vi "ReadTxBuffer.vi"(8 "error in":errorcluster, 11 "VISA Refnum in":refnum<visa-resource-name>) -> (0 "error out":errorcluster, 1 "Tx Buffer":string, 2 "Tx Buffer Len":string, 3 "VISA Refnum out":refnum<visa-resource-name>)   [LabVIEW 2020]
panel:
  out "tx_len":u32
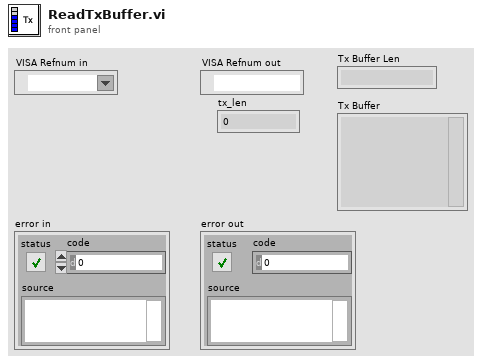
[diagram p1: front panel]
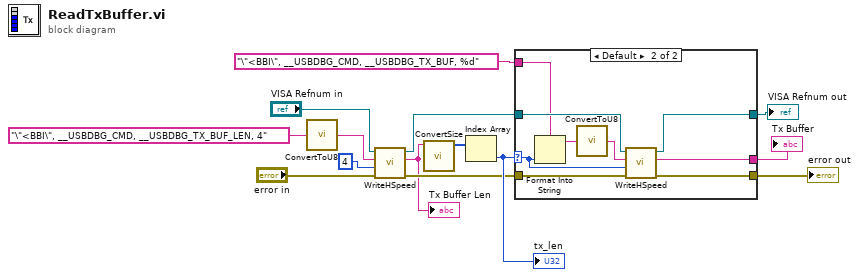
[diagram p0: block diagram]
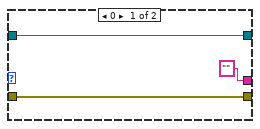
[diagram p2: hidden frame]
diagram:
  n1 = call "ConvertToU8.vi"("struct"="\"<BBI\", __USBDBG_CMD, __USBDBG_TX_BUF_LEN, 4" ("write buffer")) -> ("Binary"=w12:string)
  n2 = call "WriteHSpeed.vi"("error in"="error in", "Reply length"=4, "write buffer"=w12, "VISA Refnum in"="VISA Refnum in") -> ("error out"=w8:errorcluster, "read buffer"=w4:string, "VISA Refnum out"=w6:refnum<visa-resource-name>)  [unwired: 5 in]
  "Tx Buffer Len" <- w4
  n3 = call "ConvertSize.vi"("read buffer"=w4) -> ("size()"=w5:u32[])  [unwired: 9 in, 1 out]
  n4 = Index Array(array=w5) -> (element=w14:u32)  [unwired: 1 in]
  "tx_len" <- w14
  n5 = case shown="Default" w14 {
    selector: w14 -> [_ w19]
    tunnel: w6 -> [w17 w26]
    tunnel: w8 -> [w16 w25]
    tunnel: [w16 w24] -> w9
    tunnel: [w17 w23] -> w10
    tunnel: "\"<BBI\", __USBDBG_CMD, __USBDBG_TX_BUF, %d" ("write buffer") -> [_ w22]
    tunnel: ["" ("read buffer") w18] -> w1
    frame 0 {
    }
    frame Default {
      n6 = Format Into String(format string=w22, w19) -> (resulting string=w21:string)  [unwired: 2 in, 1 out]
      n7 = call "ConvertToU8.vi"("struct"=w21) -> ("Binary"=w20:string)
      n8 = call "WriteHSpeed.vi"("error in"=w25, "Reply length"=w19, "write buffer"=w20, "VISA Refnum in"=w26) -> ("error out"=w24:errorcluster, "read buffer"=w18:string, "VISA Refnum out"=w23:refnum<visa-resource-name>)  [unwired: 5 in]
    }
  }
  "Tx Buffer" <- w1
  "VISA Refnum out" <- w10
  "error out" <- w9
